vi "PH_ImageCoG_Plotter.Subtract Background Image.vi"(0 "i ref in":refnum<vi>, 2 "Cam Image":T1, 5 "error in (no error)":errorcluster) -> (14 "i ref out":refnum<vi>, 19 "error out":errorcluster)   [LabVIEW 2014, in "PH_ImageCoG_Plotter.lvlib"]
doc: "This VI subtracts the background image (if available). Together with the information whether this has been successful it saves the raw image and the final image to own attributes."
uses:
  PH_ImageCoG_Plotter.lvlib
  <vilib>/vision/Image Controls.llb/IMAQ Image.ctl
  PH_StatusHandler/PH_StatusHandler.Status.ctl
  PH_Common/PH_Common.lvlib
  <vilib>/vision/NI_Vision_Development_Module.lvlib
  PH_StatusHandler/PH_StatusHandler.lvlib
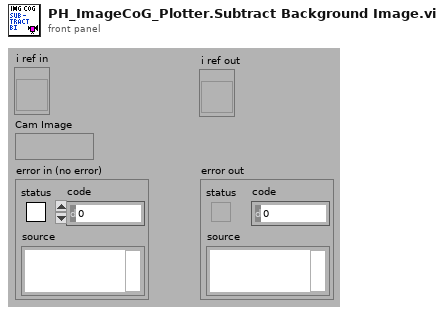
[diagram p1: front panel]
types:
  T1 = typedef "IMAQ Image.ctl" = refnum<image>
  T2 = typedef "Image Type" = u32
  T3 = typedef "PH_StatusHandler.lvlib/PH_StatusHandler.Status.ctl" = i16
  T4 = typedef "PH_ImageCoG_Plotter.lvlib/PH_ImageCoG_Plotter.i attribute.ctl" = cluster{"GUI Refs":cluster{"Delete":refnum<vi>, "Calibration status":refnum<vi>, "BI subtracted":refnum<vi>, "calc Beam Anal":refnum<vi>, "CoG - x":refnum<vi>, "CoG - y":refnum<vi>, "Type":refnum<vi>, "Center":refnum<vi>, "exp - X":refnum<vi>, "exp - Y":refnum<vi>, "Delta - X":refnum<vi>, "Delta - Y":refnum<vi>, "Available Cams":refnum<vi>, "CoG X":refnum<vi>, "CoG Y":refnum<vi>, "Delta X":refnum<vi>, "Delta Y":refnum<vi>, "Export Data":refnum<vi>, "Calibration data":refnum<vi>}, "Calibration":cluster{"Status":T3, "Calibration data":T5, "Calibration Data File":path}, "Beam Analysis":cluster{"on":bool, "exp - X":i32, "exp - Y":i32, "Type":bool, "Data":cluster{"current time":timestamp, "CoG-x":dbl, "CoG-y":dbl, "Delta-x":dbl, "Delta-y":dbl}[], "Datasets strored":i32, "Dataarray Size":i32}, "Cam instances":string[], "DIM Service Events":T6[], "Images":cluster{"Background":T1, "OP":T1, "GUI":T1}}
  T5 = typedef "PH_ImageCalibrator.lvlib/PH_ImageCalibrator.Calibration Data.ctl" = cluster{"Date":string, "Time":string, "Cam Settings":cluster{"Cam ID":string, "Gain":dbl, "Brightness":dbl, "Shutter":dbl, "Cam Error":bool, "Mode":i32}, "Background Image":cluster{"Image":dbl[][], "Image Error":bool}, "Linear Calibration":cluster{"Calibration Factor":dbl, "not mm or mrad":bool}, "Energy Calibration":cluster{"Calibration Factor":dbl, "no mJ":bool}}
  T6 = typedef "BaseProcess.lvlib/BaseProcess.event definition.ctl" = cluster{"CAEEvtDef":T7, "Data Descriptor":T8}
  T7 = typedef "CAEObj.lvlib/CAEObj.event definition.ctl" = cluster{"URL":string, "enable":bool, "ignoreResID":bool}
  T8 = typedef "BaseProcess.lvlib/BaseProcess.descriptor string definition.ctl" = string
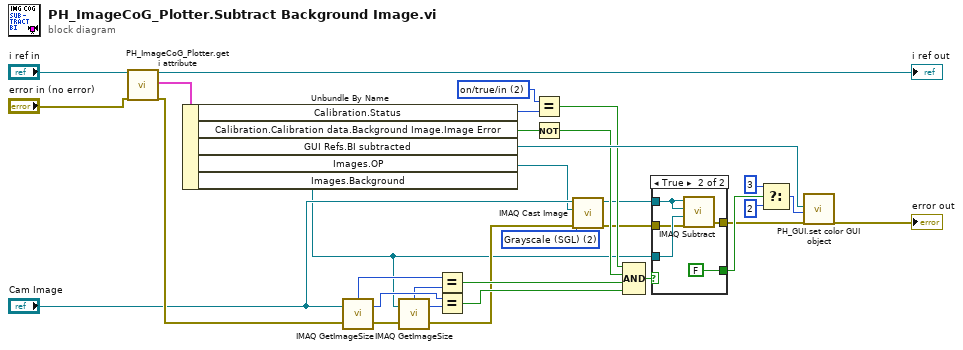
[diagram p0: block diagram]
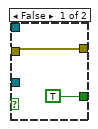
[diagram p2: hidden frame]
diagram:
  w6 = T2 2 items=["Grayscale (U8)", "Grayscale (I16)", "Grayscale (SGL)", "Complex (CSG)", "RGB (U32)", "HSL (U32)", "RGB (U64)"] ("Image Type")
  w13 = T3 2 items=["no info", "off/false/out", "on/true/in", "Failure", "Alarm", "Status 1", "Status 2", "Status 3"] ("Calibration.Status")
  n1 = call "PH_ImageCoG_Plotter.get i attribute.vi"("i ref in"="i ref in", "error in (no error)"="error in (no error)") -> ("i ref out"=→"i ref out":refnum<vi>, "i attribute"=w31:T4, "error out"=w32:errorcluster)  [unwired: 15 in]
  n2 = Unbundle By Name(w31) -> ("Calibration.Status"=w14:T3, "Calibration.Calibration data.Background Image.Image Error"=w23:bool, "GUI Refs.BI subtracted"=w12:refnum<vi>, "Images.OP"=w1:T1, "Images.Background"=w2:T1)
  n3 = call "IMAQ GetImageSize"("Image"="Cam Image", "error in (no error)"=w32) -> ("Y Resolution"=w18:i32, "X Resolution"=w16:i32, "error out"=w15:errorcluster)  [unwired: 2 in]
  n4 = call "IMAQ GetImageSize"("Image"=w2, "error in (no error)"=w15) -> ("Y Resolution"=w19:i32, "X Resolution"=w17:i32, "error out"=w9:errorcluster)  [unwired: 2 in]
  n5 = Equal?(x=w16, y=w17) -> (x = y?=w20:bool)
  n6 = Equal?(x=w18, y=w19) -> (x = y?=w21:bool)
  n7 = Equal?(x=w13, y=w14) -> (x = y?=w10:bool)
  n8 = Not(x=w23) -> (.not. x?=w11:bool)
  n9 = call "IMAQ Cast Image"("Image Type"=w6, "error in (no error)"=w9, "Image Dst"=w1, "Image Src"="Cam Image") -> ("error out"=w8:errorcluster, "Image Dst Out"=w7:T1)  [unwired: 6 in]
  n10 = Compound Arithmetic op=AND(w10, w11, w20, w21) -> (w22:bool)
  n11 = case shown="True" w22 {
    tunnel: w2 -> [_ w38]
    tunnel: w7 -> [_ w37]
    tunnel: [TRUE FALSE] -> w27
    tunnel: w8 -> [w34 w36]
    tunnel: [w34 w39] -> w5
    frame False {
    }
    frame True {
      n12 = call "IMAQ Subtract"("Image Src A"=w37, "Image Dst"=w37, "Image Src B"=w38, "error in (no error)"=w36) -> ("error out"=w39:errorcluster)  [unwired: 3 in, 1 out]
    }
  }
  n13 = Select(t=3, s=w27, f=2) -> (s? t:f=w26:i32)
  n14 = call "PH_GUI.set color GUI object.vi"("GUI object Ref"=w12, "State"=w26, "error in (no error)"=w5) -> ("error out"=→"error out":errorcluster)  [unwired: 16 in]
